vi "Measurement.Uninit.vi"(8 "error in (no error)":errorcluster, 11 "Measurement.WavelengthSweeping in":refnum<class "Measurement.WavelengthSweeping.lvclass">) -> (0 "error out":errorcluster, 3 "Measurement.WavelengthSweeping out":refnum<class "Measurement.WavelengthSweeping.lvclass">)   [LabVIEW 2017, in "Measurement.WavelengthSweeping.lvclass"]
uses:
  Measurement.WavelengthSweeping.lvclass
  OPA/OPA.lvclass
  D:/upwork/Laser Measurement Tool/Laser/project/Subsystems/Device/Device.lvclass
  OPM/OPM.lvclass
  LIA/LIA.lvclass
  SMU/SMU.lvclass
  Device/Device.lvclass
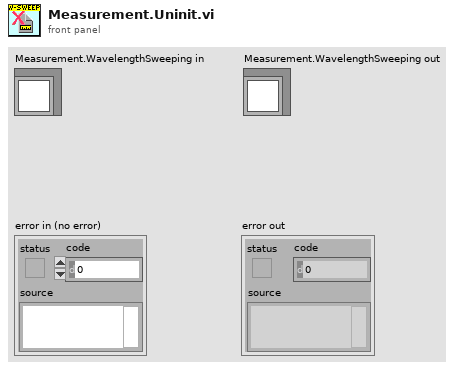
[diagram p1: front panel]
types:
  T1 = typedef "Measurement.WavelengthSweeping.lvclass/Dependencies--Cluster.ctl" = cluster{"SMU":refnum<class "SMU.lvclass">, "LIA":refnum<class "LIA.lvclass">, "OPM":refnum<class "OPM.lvclass">, "OPA":refnum<class "OPA.lvclass">}
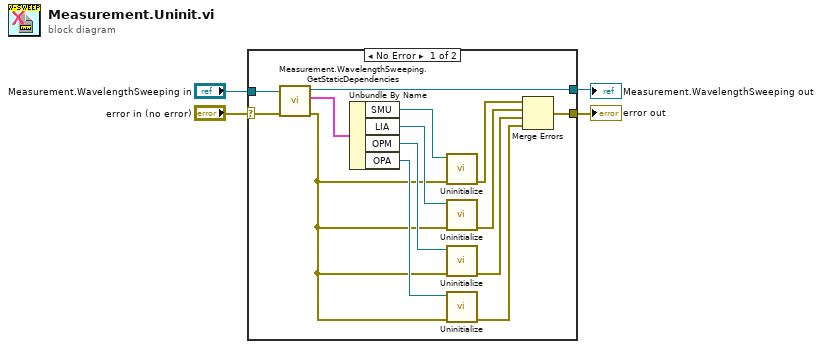
[diagram p0: block diagram]
diagram:
  n1 = case shown="No Error" "error in (no error)" {
    selector: "error in (no error)" -> [w17 w19]
    tunnel: "Measurement.WavelengthSweeping in" -> [w18 w20]
    tunnel: [w16 w20] -> w2
    tunnel: [w5 w19] -> w1
    frame No Error {
      n2 = call "Measurement.WavelengthSweeping.GetStaticDependencies.vi"("error in (no error)"=w17, "Measurement.WavelengthSweeping in"=w18) -> ("error out"=w10:errorcluster, "Dependencies"=w15:T1, "Measurement.WavelengthSweeping out"=w16:refnum<class "Measurement.WavelengthSweeping.lvclass">)  [unwired: 7 in]
      n3 = Unbundle By Name(w15) -> ("SMU"=w14:refnum<class "SMU.lvclass">, "LIA"=w13:refnum<class "LIA.lvclass">, "OPM"=w12:refnum<class "OPM.lvclass">, "OPA"=w11:refnum<class "OPA.lvclass">)
      n4 = call "Uninitialize.vi"("error in (no error)"=w10, "Device in"=w14) -> ("error out"=w9:errorcluster)  [unwired: 8 in, 1 out]
      n5 = call "Uninitialize.vi"("error in (no error)"=w10, "Device in"=w13) -> ("error out"=w8:errorcluster)  [unwired: 8 in, 1 out]
      n6 = call "Uninitialize.vi"("error in (no error)"=w10, "Device in"=w12) -> ("error out"=w7:errorcluster)  [unwired: 8 in, 1 out]
      n7 = call "Uninitialize.vi"("error in (no error)"=w10, "Device in"=w11) -> ("error out"=w6:errorcluster)  [unwired: 8 in, 1 out]
      n8 = Merge Errors(w9, w8, w7, w6) -> (w5:errorcluster)
    }
    frame Error {
    }
  }
  "error out" <- w1
  "Measurement.WavelengthSweeping out" <- w2
